vi "acceleration_quantities.vi"(1 "angular_velocity":dbl, 2 "angle_input":dbl, 3 "velocity_magnitude":dbl) -> (6 "angle_output":dbl, 7 "acceleration_magnitude":dbl, 8 "acceleration_x_component":dbl, 9 "acceleration_y_component":dbl)   [LabVIEW 2018]
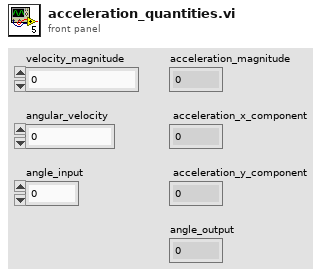
[diagram p1: front panel]
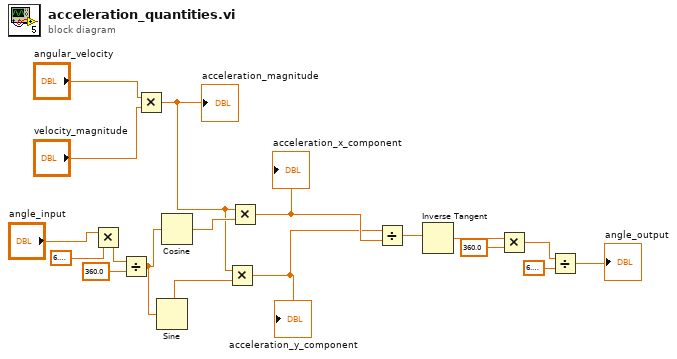
[diagram p0: block diagram]
diagram:
  n1 = Multiply(x="angle_input", y=6.283185307179586) -> (x*y=w8:dbl)
  n2 = Divide(x=w8, y=360.0) -> (x/y=w6:dbl)
  n3 = Multiply(x="angular_velocity", y="velocity_magnitude") -> (x*y=w15:dbl)
  "acceleration_magnitude" <- w15
  n4 = Sine(x=w6) -> (sin(x)=w14:dbl)
  n5 = Cosine(x=w6) -> (cos(x)=w16:dbl)
  n6 = Multiply(x=w15, y=w14) -> (x*y=w12:dbl)
  "acceleration_y_component" <- w12
  n7 = Multiply(x=w15, y=w16) -> (x*y=w13:dbl)
  "acceleration_x_component" <- w13
  n8 = Divide(x=w12, y=w13) -> (x/y=w11:dbl)
  n9 = Inverse Tangent(1:w11) -> (0:w5:dbl)
  n10 = Multiply(x=w5, y=360.0) -> (x*y=w3:dbl)
  n11 = Divide(x=w3, y=6.283185307179586) -> (x/y=→"angle_output":dbl)
